vi "总磷总氮报警信息.vi"(8 "error in (no error)":errorcluster, 11 "data in":T1) -> (0 "error out":errorcluster)   [LabVIEW 2016, in "斯坦道氨氮.lvlib"]
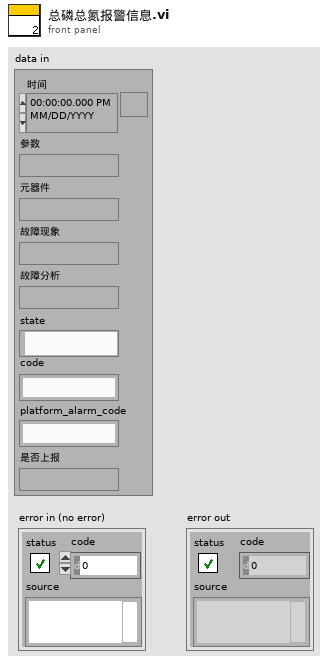
[diagram p1: front panel]
types:
  T1 = typedef "报警信息字段定义.ctl" = cluster{"时间":timestamp, "参数":string, "元器件":string, "故障现象":string, "故障分析":string, "state":string, "code":string, "platform_alarm_code":string, "是否上报":string}
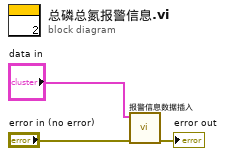
[diagram p0: block diagram]
diagram:
  n1 = call "报警信息数据插入.vi"("data"="data in", "错误输入（无错误）"="error in (no error)") -> ("错误输出"=→"error out":errorcluster)  [unwired: 8 in]
